vi "TDMS Open Err Check.vi"(5 "milliseconds to wait":u32=100, 7 "Retry attempts":i32=5, 8 "Error In":errorcluster, 10 "operation (0:open)":T1(ring), 11 "File Path Control":path) -> (0 "Error Out":errorcluster, 2 "Attempts out":i32, 3 "tdms file out":refnum<k34>)   [LabVIEW 2019]
panel:
  in  "Retry on errer numbers":i32[](array[numeric])=[8]
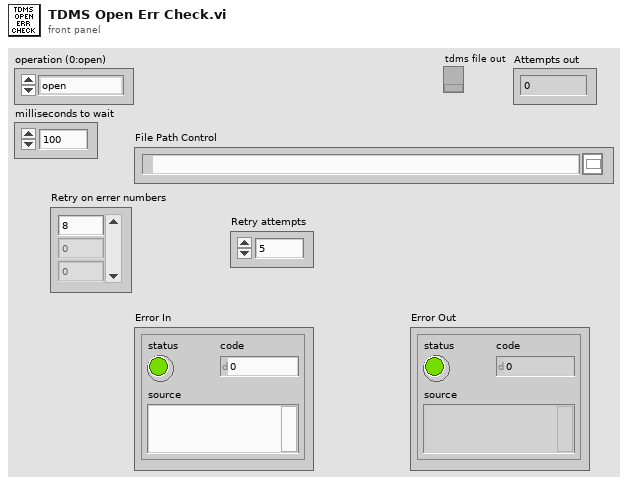
[diagram p1: front panel]
types:
  T1 = enum16{"open", "open or create", "create or replace", "create", "open (read-only)"}
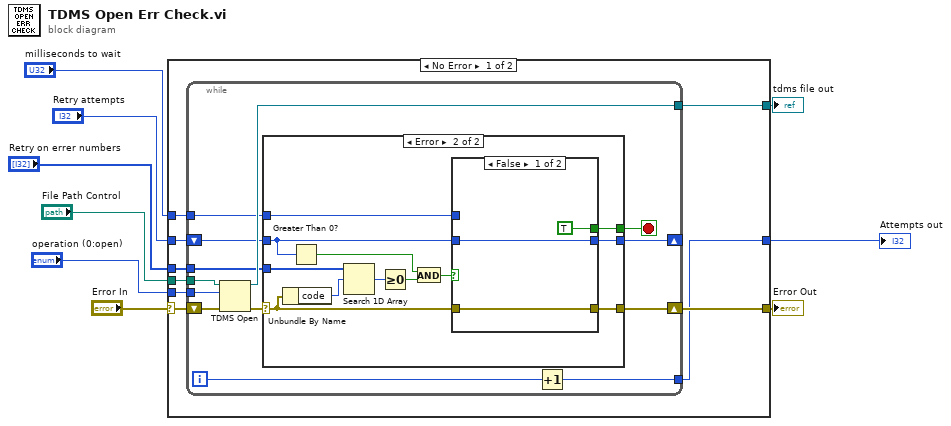
[diagram p0: block diagram]
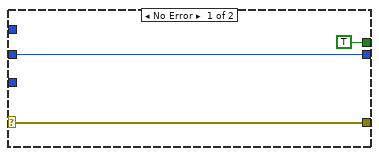
[diagram p2: hidden frame]
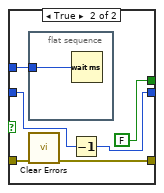
[diagram p3: hidden frame]
diagram:
  n1 = case shown="No Error" "Error In" {
    selector: "Error In" -> [w16 w57]
    tunnel: "operation (0:open)" -> [w18 _]
    tunnel: "File Path Control" -> [w17 _]
    tunnel: [w15 _] -> w6
    tunnel: [w14 w57] -> w5
    tunnel: "Retry on errer numbers" -> [w13 _]
    tunnel: "Retry attempts" -> [w12 _]
    tunnel: "milliseconds to wait" -> [w11 _]
    tunnel: [w10 _] -> w1
    frame No Error {
      n2 = while {
        tunnel: w18 -> [w31]
        tunnel: w17 -> [w29]
        tunnel: [w28] -> w15
        shift-right: [w22] -> w14
        shift-left: w16 -> [w30]
        tunnel: w13 -> [w26]
        shift-right: [w24] -> _
        shift-left: w12 -> [w25]
        tunnel: w11 -> [w23]
        tunnel: [w19] -> w10
        i -> [w20]
        stop <- w21 stop-if-true
        n3 = TDMS Open(8:w30, 10:w31, 11:w29) -> (0:w27:errorcluster, 3:w28:refnum<k34>)  [unwired: 4 in]
        n4 = case shown="Error" w27 {
          selector: w27 -> [w34 w37]
          tunnel: [w34 w36] -> w22
          tunnel: w26 -> [_ w46]
          tunnel: w25 -> [w33 w40]
          tunnel: [w33 w42] -> w24
          tunnel: w23 -> [_ w38]
          tunnel: [TRUE w35] -> w21
          frame No Error {
          }
          frame Error {
            n5 = Unbundle By Name(w37) -> ("code"=w45:i32)
            n6 = Greater Than 0?(x=w40) -> (x > 0?=w39:bool)
            n7 = Search 1D Array(1D array=w46, element=w45) -> (index of element=w44:i32)  [unwired: 1 in]
            n8 = Greater Or Equal To 0?(x=w44) -> (x >= 0?=w43:bool)
            n9 = And(x=w39, y=w43) -> (x .and. y?=w41:bool)
            n10 = case shown="False" w41 {
              tunnel: [w49 w54] -> w42
              tunnel: w40 -> [w49 w55]
              tunnel: w38 -> [_ w53]
              tunnel: w37 -> [w48 w52]
              tunnel: [w48 w51] -> w36
              tunnel: [TRUE FALSE] -> w35
              frame False {
              }
              frame True {
                n11 = flat-sequence {
                  tunnel: w53 -> [w56]
                  frame #0 {
                    n12 = Wait (ms)(milliseconds to wait=w56) -> ()  [unwired: 1 out]
                  }
                }
                n13 = call <vilib>:"Clear Errors.vi"("error in (no error)"=w52) -> ("error out"=w51:errorcluster)  [unwired: 5 in, 1 out]
                n14 = Decrement(x=w55) -> (x-1=w54:i32)
              }
            }
          }
        }
        n15 = Increment(x=w20) -> (x+1=w19:i32)
      }
    }
    frame Error {
    }
  }
  "Error Out" <- w5
  "tdms file out" <- w6
  "Attempts out" <- w1
